vi "בחירת בדיקות עבור הממסר דימום מנוע 6.vi"(0 "Enable":bool=TRUE, 5 "error in (no error)":errorcluster) -> (11 "בחר הכל":bool, 12 "בדיקת מפל מתח בין דקי הממסר תחת עומס":bool, 13 "בדיקת זמן ניתוק הממסר":bool, 14 "בדיקת זמן מיתוג הממסר":bool, 18 "OK":bool, 19 "error out":errorcluster)   [LabVIEW 2014]
doc: "Displays a standard dialog box that prompts users to enter information, such as a user name and password.\n--------------------\n\nThis Express VI is configured as follows:\n\nMessage to Display to the User:בחירת בדיקות עבור הממסר דימום מנוע\nThe inputs are: \nCheckbox: בדיקת זמן מיתוג הממסר\nCheckbox: בדיקת זמן ניתוק הממסר\nCheckbox: בדיקת מפל מתח בין דקי הממסר תחת עומס\nCheckbox: בחר הכל"
panel:
  in  "בחר הכל":bool
  in  "בדיקת מפל מתח בין דקי הממסר תחת עומס":bool
  in  "בדיקת זמן ניתוק הממסר":bool
  in  "בדיקת זמן מיתוג הממסר":bool
  in  "Cancel":bool
  in  "OK2":bool
  in  "OK1":bool
  # "בחירת בדיקות עבור הממסר דימום מנוע"
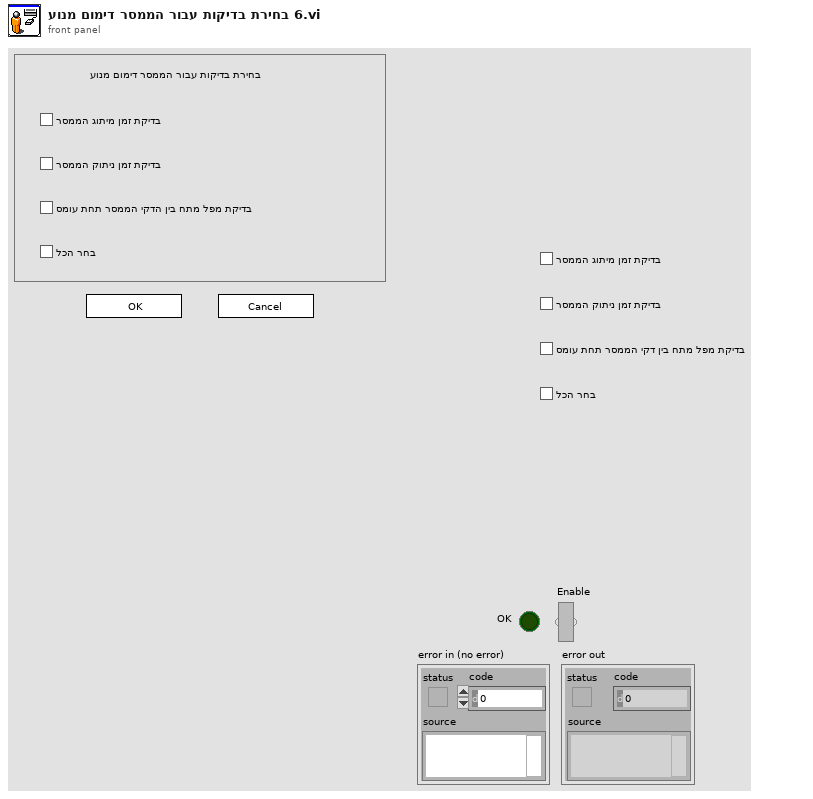
[diagram p1: front panel]
types:
  T1 = cluster{"Input Name":string, "Input Data Type":i32}[]
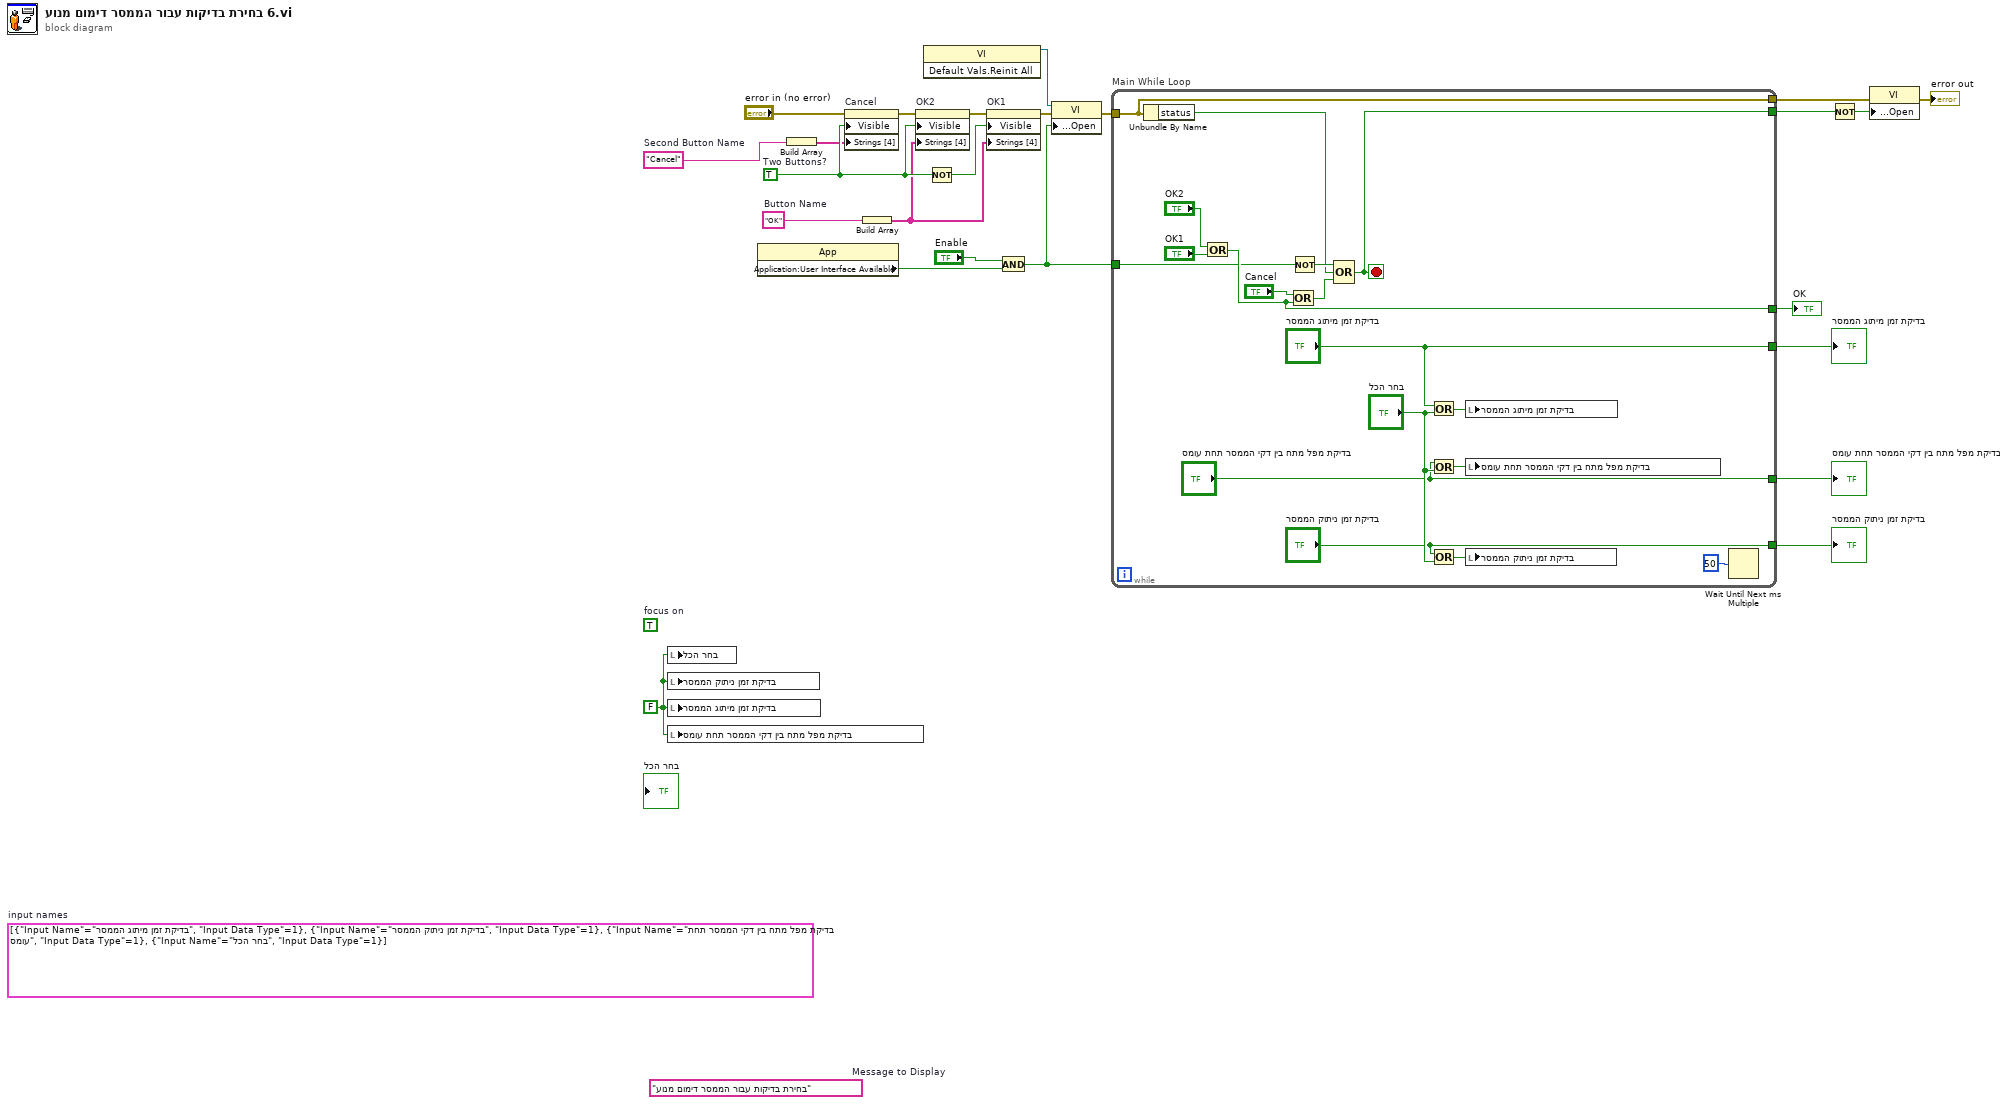
[diagram p0: block diagram]
diagram:
  (unwired) T1 [{"Input Name"="בדיקת זמן מיתוג הממסר", "Input Data Type"=1}, {"Input Name"="בדיקת זמן ניתוק הממסר", "Input Data Type"=1}, {"Input Name"="בדיקת מפל מתח בין דקי הממסר תחת עומס", "Input Data Type"=1}, {"Input Name"="בחר הכל", "Input Data Type"=1}]  # input names
  w1 = FALSE ("בחר הכל")
  (unwired) TRUE  # focus on
  w16 = "Cancel"  # Second Button Name
  w14 = "OK"  # Button Name
  (unwired) "בחירת בדיקות עבור הממסר דימום מנוע"  # Message to Display
  w24 = TRUE  # Two Buttons?
  n1 = local write "בחר הכל"(w1) -> ()
  n2 = local write "בדיקת זמן ניתוק הממסר"(w1) -> ()
  n3 = local write "בדיקת זמן מיתוג הממסר"(w1) -> ()
  n4 = local write "בדיקת מפל מתח בין דקי הממסר תחת עומס"(w1) -> ()
  n5 = property class="App"() -> ("Application:User Interface Available"=w6:bool)  [unwired: 2 in, 2 out]
  n6 = Build Array(w16) -> (w17:string[])
  n7 = property on="Cancel" class="Bool"(error in="error in (no error)", "Visible"=w24, "Strings [4]"=w17) -> (error out=w21:errorcluster)  [unwired: 1 in, 1 out]
  n8 = Build Array(w14) -> (w15:string[])
  n9 = property on="OK2" class="Bool"(error in=w21, "Visible"=w24, "Strings [4]"=w15) -> (error out=w20:errorcluster)  [unwired: 1 in, 1 out]
  n10 = invoke class="VI" method="Default Vals.Reinit All"() -> (reference out=w5:refnum<vi>)  [unwired: 3 in, 2 out]
  n11 = Not(x=w24) -> (.not. x?=w22:bool)
  n12 = property on="OK1" class="Bool"(error in=w20, "Visible"=w22, "Strings [4]"=w15) -> (error out=w13:errorcluster)  [unwired: 1 in, 1 out]
  n13 = And(x="Enable", y=w6) -> (x .and. y?=w7:bool)
  n14 = property class="VI"(reference=w5, error in=w13, "Front Panel Window:Open"=w7) -> (error out=w12:errorcluster)  [unwired: 1 out]
  n15 = while "Main While Loop" {
    tunnel: [w39] -> w23
    tunnel: w7 -> [w37]
    tunnel: [w35] -> w18
    tunnel: w12 -> [w34]
    tunnel: [w34] -> w10
    tunnel: ["בדיקת זמן מיתוג הממסר"] -> w4
    tunnel: ["בדיקת זמן ניתוק הממסר"] -> w3
    tunnel: ["בדיקת מפל מתח בין דקי הממסר תחת עומס"] -> w2
    stop <- w35 stop-if-true
    n16 = Unbundle By Name(w34) -> ("status"=w32:bool)
    n17 = Or(x="OK2", y="OK1") -> (x .or. y?=w39:bool)
    n18 = Or(x="Cancel", y=w39) -> (x .or. y?=w33:bool)
    n19 = Not(x=w37) -> (.not. x?=w36:bool)
    n20 = Compound Arithmetic op=OR(w36, w32, w33) -> (w35:bool)
    n21 = Or(x="בדיקת זמן מיתוג הממסר", y="בחר הכל") -> (x .or. y?=w28:bool)
    n22 = Or(x="בדיקת מפל מתח בין דקי הממסר תחת עומס", y="בחר הכל") -> (x .or. y?=w27:bool)
    n23 = Or(x="בדיקת זמן ניתוק הממסר", y="בחר הכל") -> (x .or. y?=w25:bool)
    n24 = local write "בדיקת זמן מיתוג הממסר"(w28) -> ()
    n25 = local write "בדיקת מפל מתח בין דקי הממסר תחת עומס"(w27) -> ()
    n26 = local write "בדיקת זמן ניתוק הממסר"(w25) -> ()
    n27 = Wait Until Next ms Multiple(millisecond multiple=u32 50) -> ()  [unwired: 1 out]
  }
  "OK" <- w23
  "בדיקת זמן מיתוג הממסר" <- w4
  "בדיקת זמן ניתוק הממסר" <- w3
  "בדיקת מפל מתח בין דקי הממסר תחת עומס" <- w2
  n28 = Not(x=w18) -> (.not. x?=w19:bool)
  n29 = property class="VI"(error in=w10, "Front Panel Window:Open"=w19) -> (error out=→"error out":errorcluster)  [unwired: 1 in, 1 out]
